vi "Extract Tetragon.vi"() -> ()   [LabVIEW 2014]
doc: "Use this template to build a VI to use as a subVI."
uses:
  <vilib>/vision/NI_Vision_Development_Module.lvlib
panel:
  out "Src":T1(plugin-control)
  out "Dst":T1(plugin-control)
  # ":: MVi Framework V1.0 ::\nAuthor:Gaoke Yang\nEmail: gaoke.yang@yahoo.com\nWeb: www.mvicontrol.com\nCopyright (C) 2015, MVI Technologies All Rights Reserved"
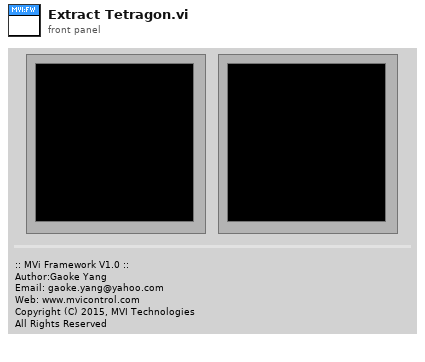
[diagram p1: front panel]
types:
  T1 = typedef "IMAQ Image.ctl" = refnum<image>
  T2 = typedef "ROI Descriptor" = cluster{"Global Rectangle":i32[], "Contours":cluster{"ID":enum32{"External", "Internal"}, "Type":u32, "Coordinates":i32[]}[]}
  T3 = cluster{"Interpolation Type":enum32{"Zero Order", "Bilinear", "Quadratic", "Cubic", "Bilinear Fixed"}, "Destination Width":u32, "Destination Height":u32, "Fill Value":sgl}
  T4 = typedef "Image Type" = u32
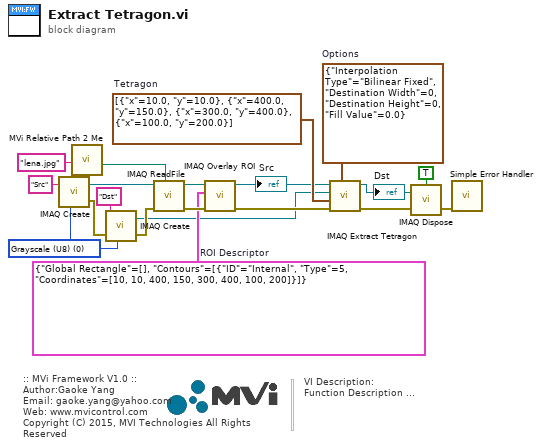
[diagram p0: block diagram]
diagram:
  w4 = T2 {"Global Rectangle"=[], "Contours"=[{"ID"=enum."Internal", "Type"=5, "Coordinates"=[10, 10, 400, 150, 300, 400, 100, 200]}]}  # ROI Descriptor
  w5 = cluster{"x":sgl, "y":sgl}[] [{"x"=10.0, "y"=10.0}, {"x"=400.0, "y"=150.0}, {"x"=300.0, "y"=400.0}, {"x"=100.0, "y"=200.0}]  # Tetragon
  w10 = T3 {"Interpolation Type"=enum."Bilinear Fixed", "Destination Width"=0, "Destination Height"=0, "Fill Value"=0.0}  # Options
  w14 = T4 0 items=["Grayscale (U8)", "Grayscale (I16)", "Grayscale (SGL)", "Complex (CSG)", "RGB (U32)", "HSL (U32)", "RGB (U64)", "Grayscale (U16)"] ("Image Type")
  # "VI Description:\nFunction Description ..."
  # ":: MVi Framework V1.0 ::\nAuthor:Gaoke Yang\nEmail: gaoke.yang@yahoo.com\nWeb: www.mvicontrol.com\nCopyright (C) 2015, MVI Technologies All Rights Reserved"
  n1 = call "IMAQ Create"("Image Name"="Src" ("name or relative path"), "Image Type"=w14) -> ("New Image"=w11:T1, "error out"=w13:errorcluster)  [unwired: 2 in, 1 out]
  n2 = call "MVi Relative Path 2 Me.vi"("Relative Path"="lena.jpg" ("name or relative path")) -> ("Appended Dir"=w16:path)  [unwired: 5 in, 1 out]
  n3 = call "IMAQ Create"("Image Name"="Dst" ("name or relative path"), "Image Type"=w14, "error in (no error)"=w13) -> ("New Image"=w2:T1, "error out"=w12:errorcluster)  [unwired: 1 in, 1 out]
  n4 = call "IMAQ ReadFile"("File Path"=w16, "error in (no error)"=w12, "Image"=w11) -> ("error out"=w6:errorcluster, "Image Out"=w7:T1)  [unwired: 4 in, 3 out]
  n5 = call "IMAQ Overlay ROI"("error in (no error)"=w6, "ROI Descriptor"=w4, "Image"=w7) -> ("error out"=w3:errorcluster, "Image Out"=w1:T1)  [unwired: 7 in]
  "Src" <- w1
  n6 = call-poly "IMAQ Extract Tetragon"("Options"=w10, "error in (no error)"=w3, "Tetragon"=w5, "Image Dst"=w2, "Image Src"=w1) -> ("error out"=w9:errorcluster, "Image Dst Out"=w8:T1)  [unwired: 5 in]
  "Dst" <- w8
  n7 = call "IMAQ Dispose"("All Images? (No)"=TRUE, "Image"=w8, "error in (no error)"=w9) -> ("error out"=w17:errorcluster)  [unwired: 3 out]
  n8 = call <vilib>:"Simple Error Handler.vi"("error in (no error)"=w17) -> ()  [unwired: 1 in, 8 out]
